vi "计算系数.vi"(8 "量程A":dbl, 9 "量程B":dbl, 10 "传感器输出范围B":dbl=5.0, 11 "传感器输出范围A":dbl) -> (1 "系数":dbl[](array[numeric]), 2 "b":dbl, 3 "k":dbl)   [LabVIEW 2016]
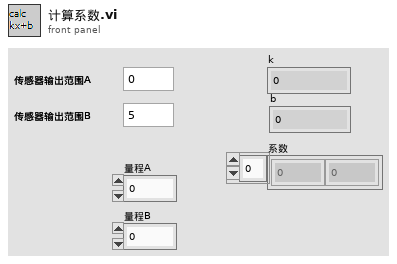
[diagram p1: front panel]
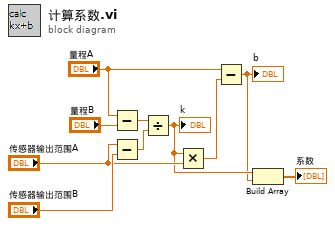
[diagram p0: block diagram]
diagram:
  n1 = Subtract(x="量程A", y="量程B") -> (x-y=w8:dbl)
  n2 = Subtract(x="传感器输出范围A", y="传感器输出范围B") -> (x-y=w7:dbl)
  n3 = Divide(x=w8, y=w7) -> (x/y=w3:dbl)
  "k" <- w3
  n4 = Multiply(x=w3, y="传感器输出范围A") -> (x*y=w4:dbl)
  n5 = Subtract(x="量程A", y=w4) -> (x-y=w2:dbl)
  "b" <- w2
  n6 = Build Array(w3, w2) -> (→"系数":dbl[])
